vi "Menu - Tags Delete App__SubVIs-某型振动实验台测试系统.vi"(1 "menu tags in":string[](array[string])) -> (0 "menu tags out":string[](array[string]))   [LabVIEW 2011]
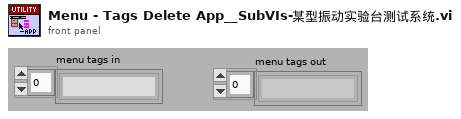
[diagram p1: front panel]
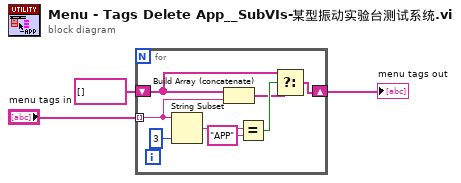
[diagram p0: block diagram]
diagram:
  n1 = for {
    shift-right: [w4] -> w3
    shift-left: string[] [] ("submenu tags") -> [w5]
    tunnel: "menu tags in" -> [w6] mode=indexing
    n2 = String Subset(string=w6, length (rest)=3 ("length (rest)")) -> (substring=w10:string)  [unwired: 1 out]
    n3 = Build Array (concatenate)(w5, w6) -> (w7:string[])
    n4 = Equal?(x=w10, y="APP") -> (x = y?=w8:bool)
    n5 = Select(t=w5, s=w8, f=w7) -> (s? t:f=w4:string[])
  }
  "menu tags out" <- w3
